vi "Print List of Hardware (String).vi"(9 "Device Names":string[](array[string])) -> (3 "String":string)   [LabVIEW 2016, in "Controller Actor.lvlib" / "Controller.lvclass"]
uses:
  <userlib>/Common Components/Controller/Controller.lvclass
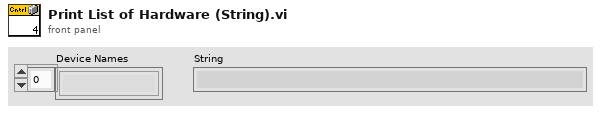
[diagram p1: front panel]
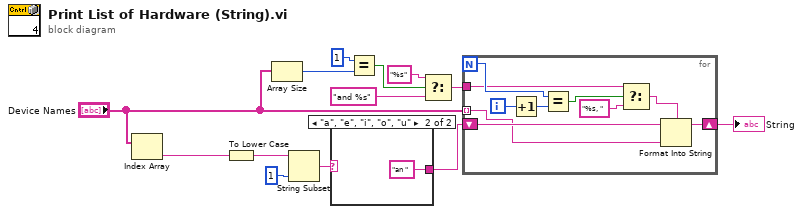
[diagram p0: block diagram]
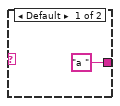
[diagram p2: hidden frame]
diagram:
  n1 = Index Array(array="Device Names") -> (element=w1:string)  [unwired: 1 in]
  n2 = To Lower Case(string=w1) -> (all lower case string=w5:string)
  n3 = Array Size(array="Device Names") -> (size(s)=w12:i32)
  n4 = String Subset(string=w5, length (rest)=1 ("length (rest)")) -> (substring=w3:string)  [unwired: 1 in]
  n5 = case shown="\"a\", \"e\", \"i\", \"o\", \"u\"" w3 {
    tunnel: ["a " "an "] -> w2
    frame Default {
    }
    frame "a", "e", "i", "o", "u" {
    }
  }
  n6 = Equal?(x=1, y=w12) -> (x = y?=w10:bool)
  n7 = Select(t="%s", s=w10, f="and %s" ("format string")) -> (s? t:f=w8:string)
  n8 = for {
    N -> [w20]
    shift-right: [w25] -> w13
    shift-left: w2 -> [w24]
    tunnel: "Device Names" -> [w23] mode=indexing
    tunnel: w8 -> [w16]
    i -> [w22]
    n9 = Increment(x=w22) -> (x+1=w21:i32)
    n10 = Equal?(x=w20, y=w21) -> (x = y?=w19:bool)
    n11 = Select(t=w16, s=w19, f="%s, " ("format string")) -> (s? t:f=w17:string)
    n12 = Format Into String(format string=w17, initial string=w24, w23) -> (resulting string=w25:string)  [unwired: 1 in, 1 out]
  }
  "String" <- w13
